vi "Calculate Message Class Path.vi"(10 "Method VI Name":string, 11 "Actor Class Path":path) -> (2 "Message Class Path":path)   [LabVIEW 2020, in "Message Maker.lvlib"]
uses:
  Message Maker.lvlib
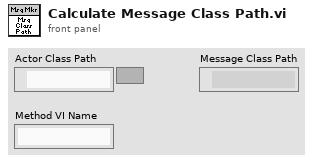
[diagram p1: front panel]
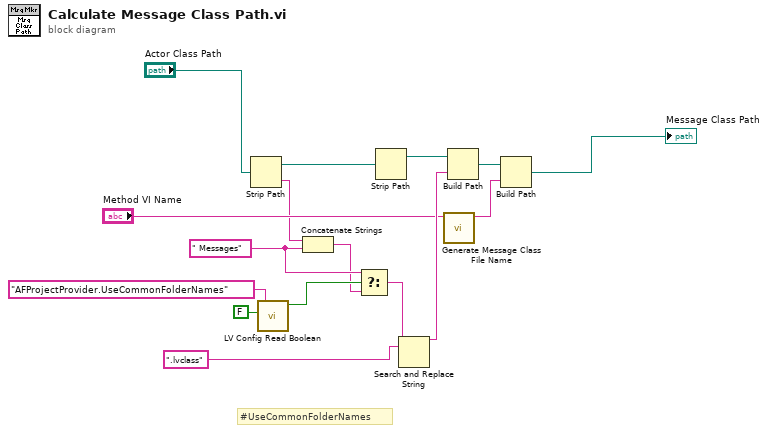
[diagram p0: block diagram]
diagram:
  w3 = " Messages" ("string")
  # "#UseCommonFolderNames"
  n1 = Strip Path(path="Actor Class Path") -> (stripped path=w8:path, name=w13:string)
  n2 = call <resource>:"LV Config Read Boolean.vi"("default value"=FALSE, "key"="AFProjectProvider.UseCommonFolderNames") -> ("value"=w4:bool)  [unwired: 3 in, 2 out]
  n3 = Concatenate Strings(w13, w3) -> (w1:string)
  n4 = Select(t=w3, s=w4, f=w1) -> (s? t:f=w2:string)
  n5 = Strip Path(path=w8) -> (stripped path=w12:path)  [unwired: 1 out]
  n6 = Search and Replace String(input string=w2, search string=".lvclass" ("string")) -> (result string=w15:string)  [unwired: 6 in, 3 out]
  n7 = call "Generate Message Class File Name.vi"("Target Method"="Method VI Name") -> ("Msg Class File Name"=w10:string)  [unwired: 10 in]
  n8 = Build Path(base path=w12, name or relative path=w15) -> (appended path=w11:path)
  n9 = Build Path(base path=w11, name or relative path=w10) -> (appended path=→"Message Class Path":path)
